vi "Tosca-Send Abort.vi"   [LabVIEW 2020]
uses:
  Tosca-Message.ctl
  Tosca-Message Action.ctl
types:
  T1 = typedef "Tosca-Message Action.ctl" = enum16{"None", "Update", "Events", "Timeout", "Error", "Abort"}
  T2 = typedef "Tosca-Message.ctl" = cluster{"Action":T1, "Time":u32, "State":i32, "Events":bool[], "Error":errorcluster}
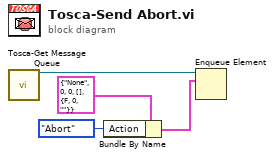
[diagram p0: block diagram]
diagram:
  n1 = call "Tosca-Get Message Queue.vi"() -> ("Message Queue"=w4:refnum<queue>)  [unwired: 14 in, 1 out]
  n2 = Bundle By Name(cluster=T2 {"Action"=enum."None", "Time"=0, "State"=0, "Events"=[], "Error"={"status"=FALSE, "code"=0, "source"=""}} ("element"), "Action"=Tosca-Message_Action."Abort") -> (w1:T2)
  n3 = Enqueue Element(queue=w4, element=w1) -> ()  [unwired: 2 in, 3 out]
